vi "前2 (子VI).vi"(10 "x":dbl) -> (2 "簇 个位":T1, 3 "簇 十位":T1)   [LabVIEW 2020]
panel:
  out "簇":T2
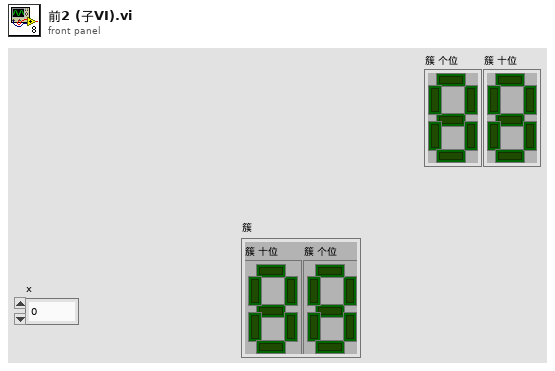
[diagram p1: front panel]
types:
  T1 = cluster{"布尔":bool, "布尔 2":bool, "布尔 3":bool, "布尔 4":bool, "布尔 5":bool, "布尔 6":bool, "布尔 7":bool}
  T2 = cluster{"簇 十位":cluster{"布尔":bool, "布尔 2":bool, "布尔 3":bool, "布尔 4":bool, "布尔 5":bool, "布尔 6":bool, "布尔 7":bool}, "簇 个位 ":cluster{"布尔":bool, "布尔 2":bool, "布尔 3":bool, "布尔 4":bool, "布尔 5":bool, "布尔 6":bool, "布尔 7":bool}}
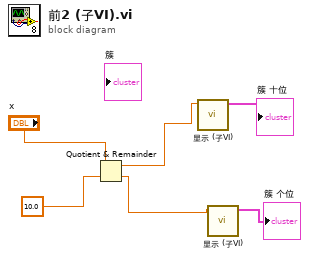
[diagram p0: block diagram]
diagram:
  n1 = Quotient & Remainder(x="x", y=10.0) -> (x-y*floor(x/y)=w3:dbl, floor(x/y)=w4:dbl)
  n2 = call "显示 (子VI).vi"("数值"=w3) -> ("簇 个位"=→"簇 十位":T1)  [unwired: 9 in]
  n3 = call "显示 (子VI).vi"("数值"=w4) -> ("簇 个位"=→"簇 个位":T1)  [unwired: 9 in]
